vi "Dispose.vi"(8 "error in (no error)":errorcluster caption="错误输入（无错误）", 11 "Mail 输入":refnum<class "Email.lvclass"> caption="DNL_LabVIEW Object in") -> (0 "error out":errorcluster caption="错误输出", 3 "Mail 输出":refnum<class "Email.lvclass"> caption="DNL_LabVIEW Object out")   [LabVIEW 2012, in "Email.lvclass"]
uses:
  Email.lvclass
  Email.lvclass/Email.ctl
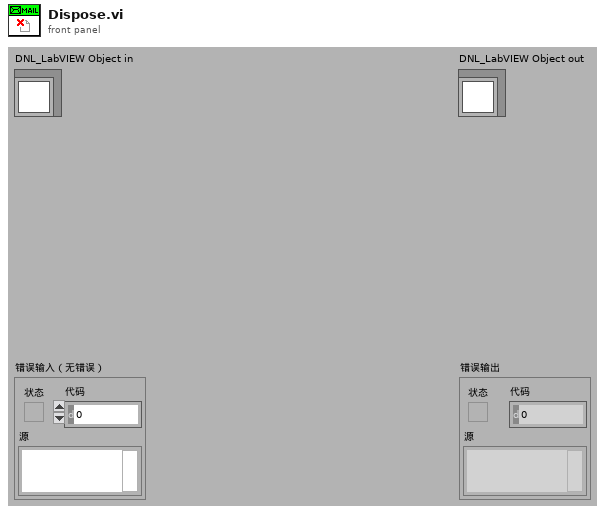
[diagram p1: front panel]
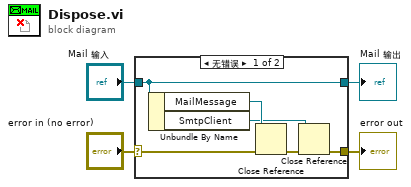
[diagram p0: block diagram]
diagram:
  n1 = case shown="无错误" "error in (no error)" {
    selector: "error in (no error)" -> [w7 w12]
    tunnel: [w5 w12] -> w3
    tunnel: [w10 w11] -> w1
    tunnel: "Mail 输入" -> [w10 w11]
    frame No Error {
      n2 = Unbundle By Name(w10) -> ("MailMessage"=w9:refnum<k24>, "SmtpClient"=w8:refnum<k24>)
      n3 = Close Reference(reference=w9, error in (no error)=w7) -> (error out=w6:errorcluster)
      n4 = Close Reference(reference=w8, error in (no error)=w6) -> (error out=w5:errorcluster)
    }
    frame Error {
    }
  }
  "error out" <- w3
  "Mail 输出" <- w1
